vi "host.vi"() -> ()   [LabVIEW 2018]
uses:
  dll/NewTmMdsSaveLoad.dll
  epics dll/JtextEPICSforNewTM.dll
  <vilib>/rvi/interface/nirviOpenFPGA/nirviOpenFPGA.xnode
  <vilib>/FPGAPlugInAG/PCI-7813R/niLvFpga_Open_PCI-7813R.vi
  <vilib>/rvi/interface/common/dynamic/niFpgaDynamicAddResources.vi
  <vilib>/rvi/interface/nirviReadWriteControl/nirviReadWriteControl.xnode
  NiFpgaLv.dll
  <vilib>/Utility/error.llb/Error Cluster From Error Code.vi
  <vilib>/rvi/interface/Simulation/niFpgaSimulationCallBeginRW.vi
  <vilib>/rvi/errors/niLvFpgaAdjustHostInterfaceError.vi
  <vilib>/rvi/interface/nirviMethod/nirviMethod.xnode
  <vilib>/FPGAPlugInAG/Dynamic/niLvFpga_Run_Dynamic.vi
panel:
  in  "have run":enum32{"选项卡 1", "选项卡 2", "选项卡 3"}(tab)
  out "hr 1":T1
  out "hr 2":T2
  out "hr 3":T3
  in  "默认night":T1
  in  "禁用Shutup":bool
  in  "禁用Trigger":bool
  in  "be running":enum32{"选项卡 1", "选项卡 2", "选项卡 3"}(tab)
  out "lvht 1":T1
  out "lvht 2":T2
  out "lvht 3":T3
  out "act 3":bool[](array[boolean])
  out "act 2":bool[](array[boolean])
  out "act 1":bool[](array[boolean])
  out "width 3":i32[](array[numeric])
  out "begin 3":i32[](array[numeric])
  out "width 2":i32[](array[numeric])
  out "width 1":i32[](array[numeric])
  out "begin 2":i32[](array[numeric])
  out "begin 1":i32[](array[numeric])
  in  "Abort":bool
  in  "Apply":bool
  in  "最大通道数量":enum16{"96", "192", "288"}(ring)
  out "最大值":u32
  out "width":i32[](array[numeric])
  out "begin":i32[](array[numeric])
  in  "Debug":bool
  in  "Config":bool
  in  "Go":bool
  out "pv=0":bool
  out "ab":bool
  out "ShutUp":bool
  out "Ready":bool
  out "stop":bool
  out "running":bool
  out "TM state":string
  in  "pvName":string="ST:GLOBAL:CTRLSTATE"
  out "错误输出":errorcluster
  out "pv失败":bool
  in  "PV":i32=-666
  in  "Shot Number":i32
  in  "tag":string="\\NEW_TM_SET"
  in  "tree name":string="jtext"
  in  "host ip":string="192.168.1.1"
  in  "修改":T4
  in  "Mdsplus":bool
  in  "Import":path
  in  "Import":bool
  in  "Export Base Path":path
  in  "Export name":string
  in  "初始化":bool
  in  "export":bool
  in  "修改":bool
  in  "修改通道选择":enum16{"1", "2", "3", "4"}(ring)
  out "act":bool[](array[boolean])
  out "title":string[](array[string])
  out "start":dbl[](array[numeric])
  out "lenght":dbl[](array[numeric])
  out "detail":string[](array[string])
  # "be running"
  # "have run"
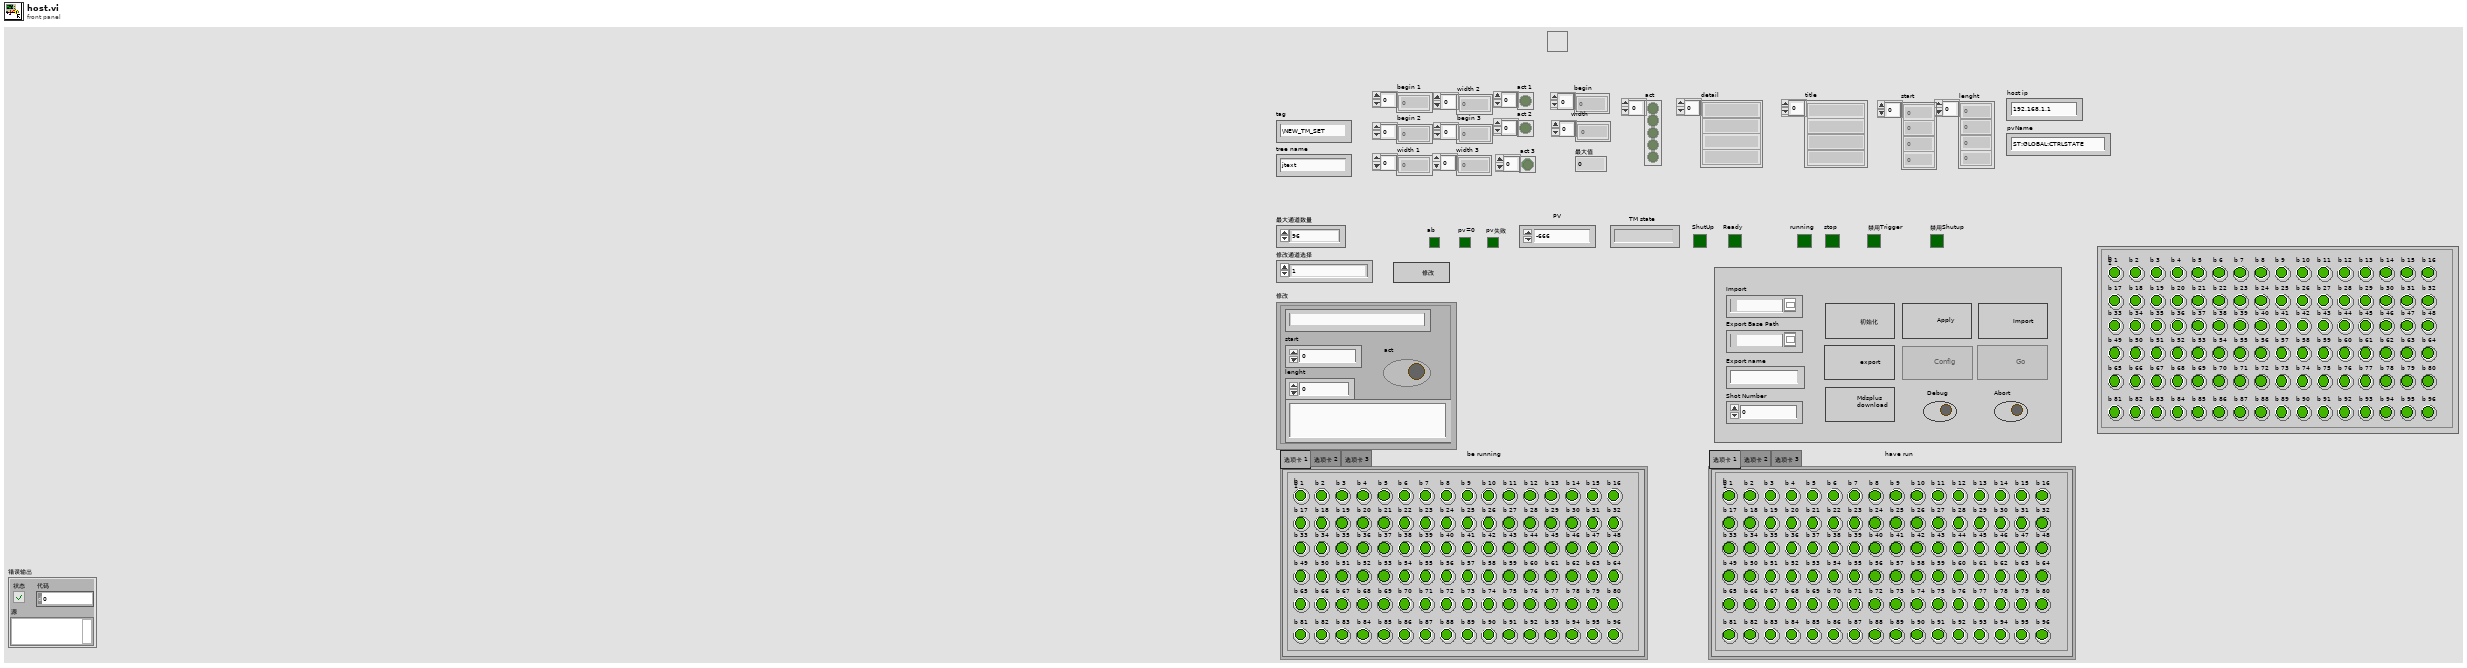
[diagram p1: front panel]
types:
  T1 = cluster{"b 1":bool, "b 2":bool, "b 3":bool, "b 4":bool, "b 5":bool, "b 6":bool, "b 7":bool, "b 8":bool, "b 9":bool, "b 10":bool, "b 11":bool, "b 12":bool, "b 13":bool, "b 14":bool, "b 15":bool, "b 16":bool, "b 17":bool, "b 18":bool, "b 19":bool, "b 20":bool, "b 21":bool, "b 22":bool, "b 23":bool, "b 24":bool, "b 25":bool, "b 26":bool, "b 27":bool, "b 28":bool, "b 29":bool, "b 30":bool, "b 31":bool, "b 32":bool, "b 33":bool, "b 34":bool, "b 35":bool, "b 36":bool, "b 37":bool, "b 38":bool, "b 39":bool, "b 40":bool, "b 41":bool, "b 42":bool, "b 43":bool, "b 44":bool, "b 45":bool, "b 46":bool, "b 47":bool, "b 48":bool, "b 49":bool, "b 50":bool, "b 51":bool, "b 52":bool, "b 53":bool, "b 54":bool, "b 55":bool, "b 56":bool, "b 57":bool, "b 58":bool, "b 59":bool, "b 60":bool, "b 61":bool, "b 62":bool, "b 63":bool, "b 64":bool, "b 65":bool, "b 66":bool, "b 67":bool, "b 68":bool, "b 69":bool, "b 70":bool, "b 71":bool, "b 72":bool, "b 73":bool, "b 74":bool, "b 75":bool, "b 76":bool, "b 77":bool, "b 78":bool, "b 79":bool, "b 80":bool, "b 81":bool, "b 82":bool, "b 83":bool, "b 84":bool, "b 85":bool, "b 86":bool, "b 87":bool, "b 88":bool, "b 89":bool, "b 90":bool, "b 91":bool, "b 92":bool, "b 93":bool, "b 94":bool, "b 95":bool, "b 96":bool}
  T2 = cluster{"b 97":bool, "b 98":bool, "b 99":bool, "b 100":bool, "b 101":bool, "b 102":bool, "b 103":bool, "b 104":bool, "b 105":bool, "b 106":bool, "b 107":bool, "b 108":bool, "b 109":bool, "b 110":bool, "b 111":bool, "b 112":bool, "b 113":bool, "b 114":bool, "b 115":bool, "b 116":bool, "b 117":bool, "b 118":bool, "b 119":bool, "b 120":bool, "b 121":bool, "b 122":bool, "b 123":bool, "b 124":bool, "b 125":bool, "b 126":bool, "b 127":bool, "b 128":bool, "b 129":bool, "b 130":bool, "b 131":bool, "b 132":bool, "b 133":bool, "b 134":bool, "b 135":bool, "b 136":bool, "b 137":bool, "b 138":bool, "b 139":bool, "b 140":bool, "b 141":bool, "b 142":bool, "b 143":bool, "b 144":bool, "b 145":bool, "b 146":bool, "b 147":bool, "b 148":bool, "b 149":bool, "b 150":bool, "b 151":bool, "b 152":bool, "b 153":bool, "b 154":bool, "b 155":bool, "b 156":bool, "b 157":bool, "b 158":bool, "b 159":bool, "b 160":bool, "b 161":bool, "b 162":bool, "b 163":bool, "b 164":bool, "b 165":bool, "b 166":bool, "b 167":bool, "b 168":bool, "b 169":bool, "b 170":bool, "b 171":bool, "b 172":bool, "b 173":bool, "b 174":bool, "b 175":bool, "b 176":bool, "b 177":bool, "b 178":bool, "b 179":bool, "b 180":bool, "b 181":bool, "b 182":bool, "b 183":bool, "b 184":bool, "b 185":bool, "b 186":bool, "b 187":bool, "b 188":bool, "b 189":bool, "b 190":bool, "b 191":bool, "b 192":bool}
  T3 = cluster{"b 193":bool, "b 194":bool, "b 195":bool, "b 196":bool, "b 197":bool, "b 198":bool, "b 199":bool, "b 200":bool, "b 201":bool, "b 202":bool, "b 203":bool, "b 204":bool, "b 205":bool, "b 206":bool, "b 207":bool, "b 208":bool, "b 209":bool, "b 210":bool, "b 211":bool, "b 212":bool, "b 213":bool, "b 214":bool, "b 215":bool, "b 216":bool, "b 217":bool, "b 218":bool, "b 219":bool, "b 220":bool, "b 221":bool, "b 222":bool, "b 223":bool, "b 224":bool, "b 225":bool, "b 226":bool, "b 227":bool, "b 228":bool, "b 229":bool, "b 230":bool, "b 231":bool, "b 232":bool, "b 233":bool, "b 234":bool, "b 235":bool, "b 236":bool, "b 237":bool, "b 238":bool, "b 239":bool, "b 240":bool, "b 241":bool, "b 242":bool, "b 243":bool, "b 244":bool, "b 245":bool, "b 246":bool, "b 247":bool, "b 248":bool, "b 249":bool, "b 250":bool, "b 251":bool, "b 252":bool, "b 253":bool, "b 254":bool, "b 255":bool, "b 256":bool, "b 257":bool, "b 258":bool, "b 259":bool, "b 260":bool, "b 261":bool, "b 262":bool, "b 263":bool, "b 264":bool, "b 265":bool, "b 266":bool, "b 267":bool, "b 268":bool, "b 269":bool, "b 270":bool, "b 271":bool, "b 272":bool, "b 273":bool, "b 274":bool, "b 275":bool, "b 276":bool, "b 277":bool, "b 278":bool, "b 279":bool, "b 280":bool, "b 281":bool, "b 282":bool, "b 283":bool, "b 284":bool, "b 285":bool, "b 286":bool, "b 287":bool, "b 288":bool}
  T4 = cluster{"title":string, "act":bool, "start":dbl, "lenght":dbl, "detail":string}
  T5 = enum16{"open", "open or create", "create or replace", "create", "open (read-only)"}
  T6 = cluster{string[], bool[], dbl[], dbl[], string[]}
  T7 = enum16{"open", "replace", "create", "open or create", "replace or create", "replace or create with confirmation"}
  T8 = cluster{"字符串":string, "act":bool, "start":dbl, "lenght":dbl, "详细信息":string}
  T9 = enum8{"Enabled", "Disabled", "Disabled and Grayed Out"}
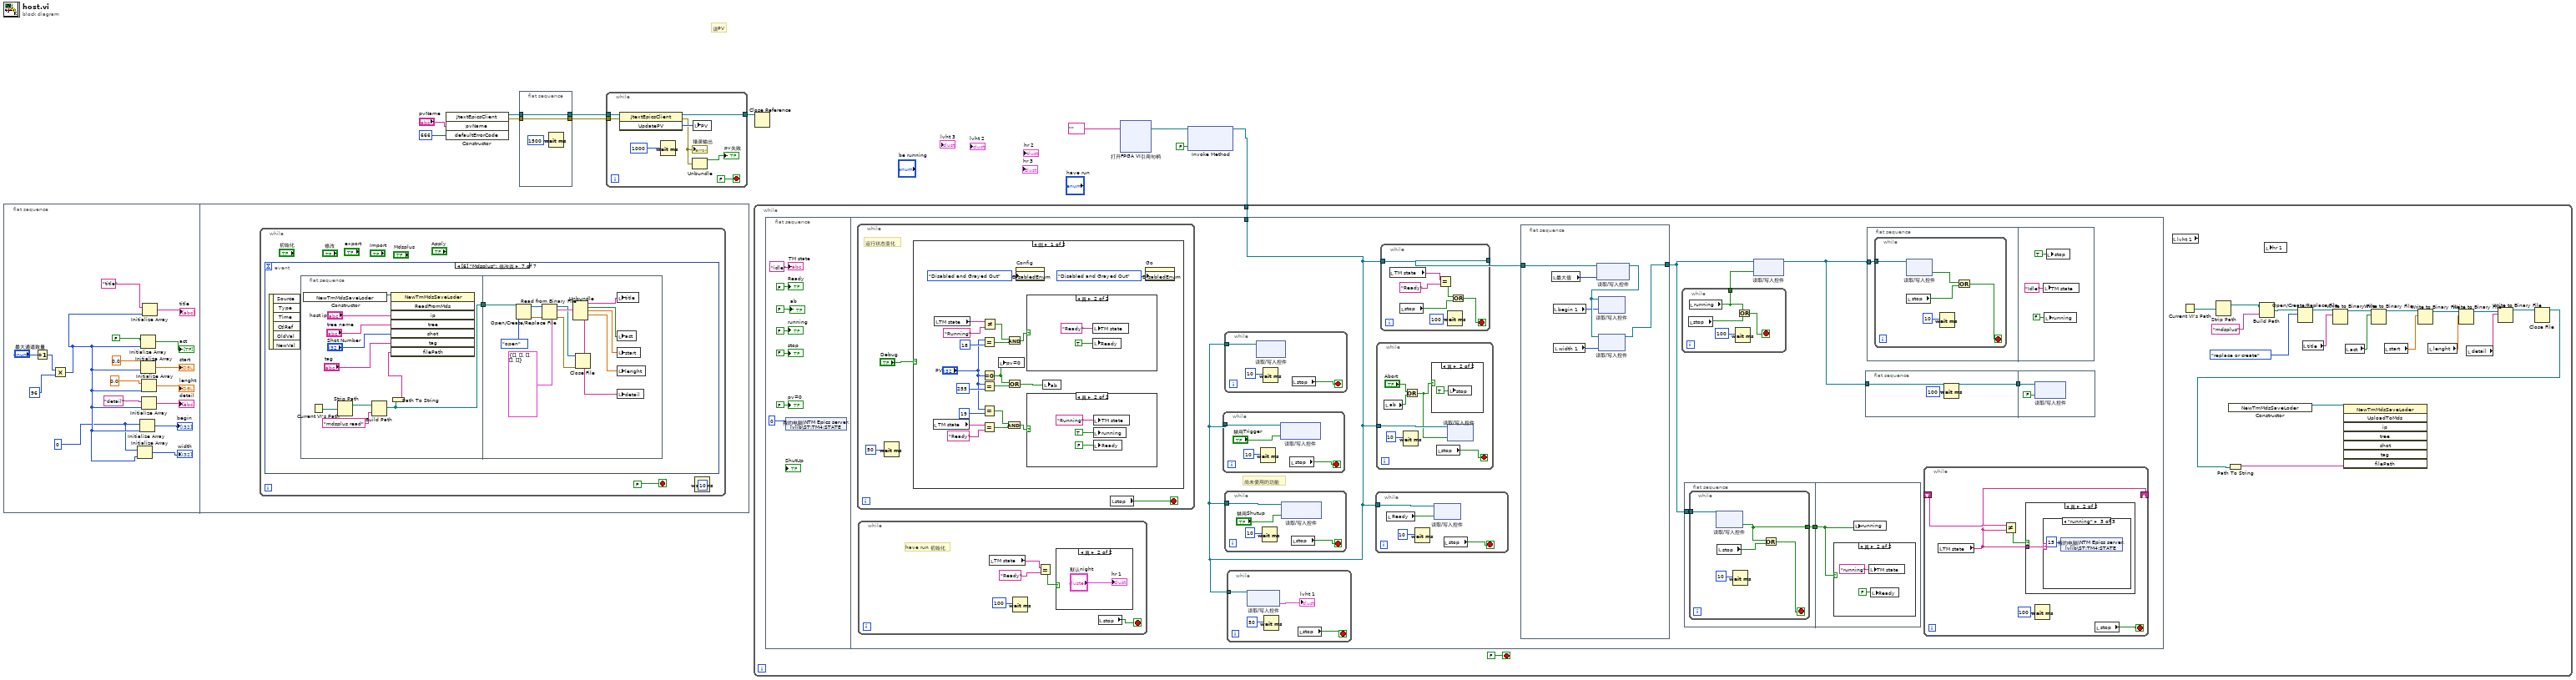
[diagram p0: block diagram]
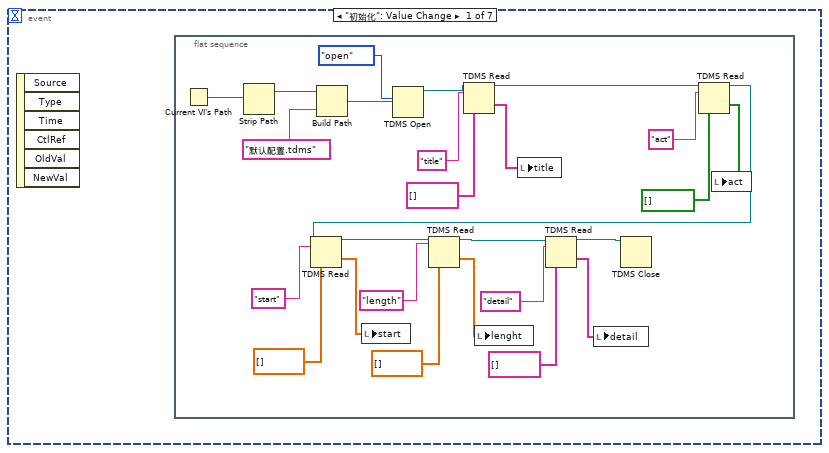
[diagram p2: hidden frame]
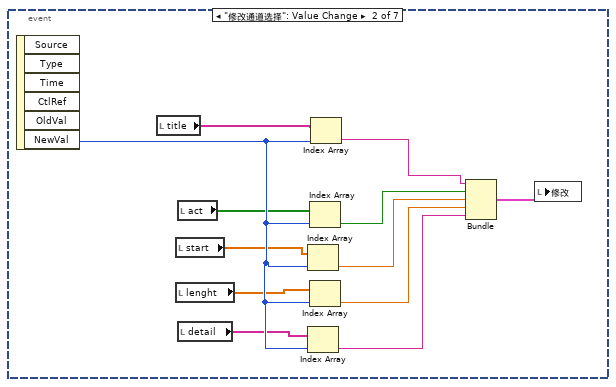
[diagram p3: hidden frame]
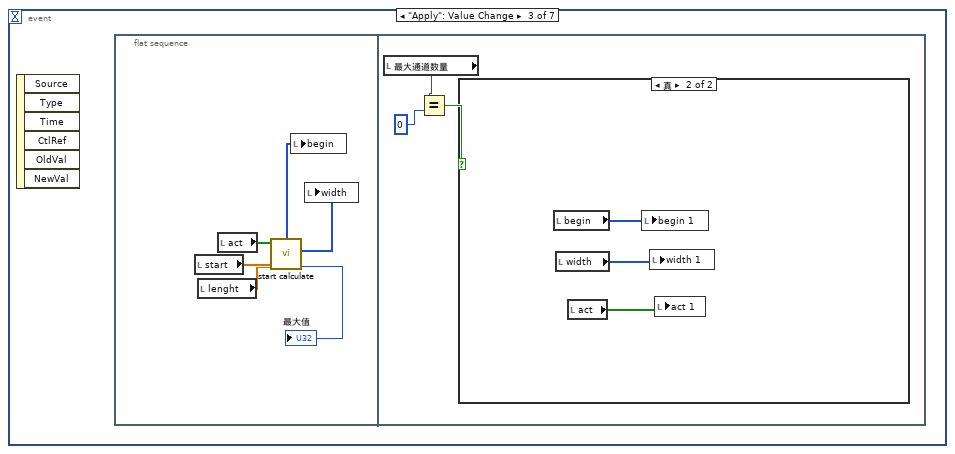
[diagram p4: hidden frame]
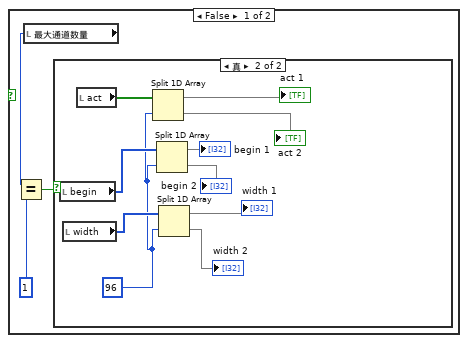
[diagram p5: hidden frame]
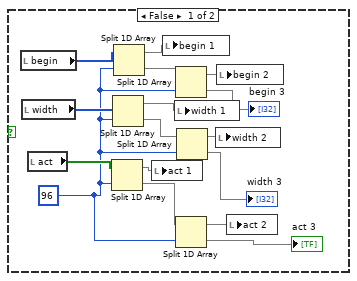
[diagram p6: hidden frame]
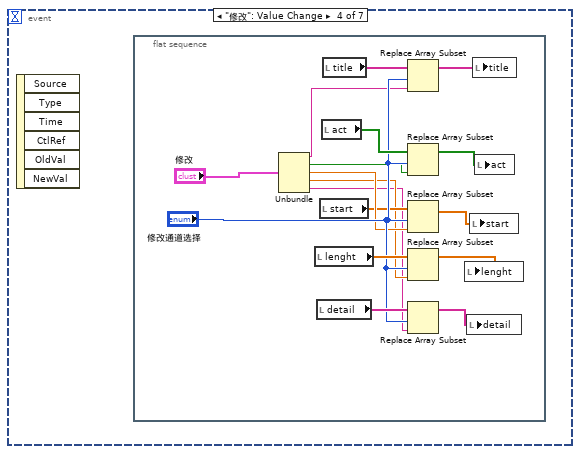
[diagram p7: hidden frame]
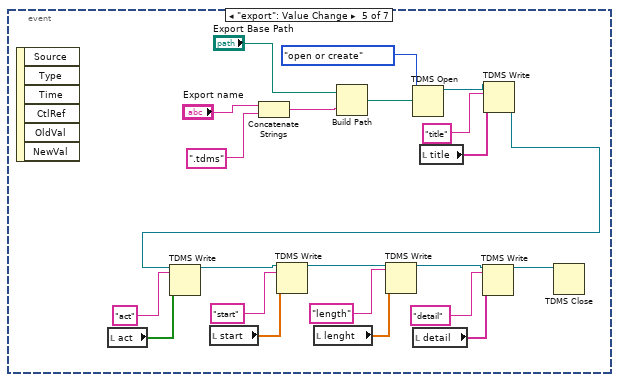
[diagram p8: hidden frame]
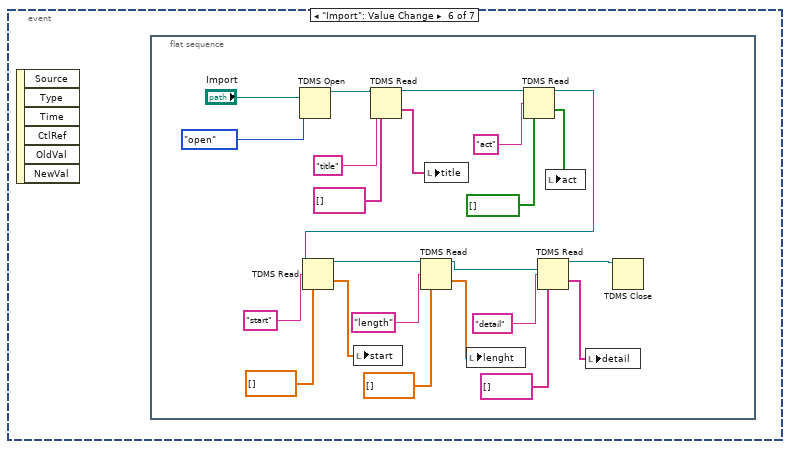
[diagram p9: hidden frame]
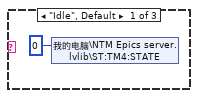
[diagram p11: hidden frame]
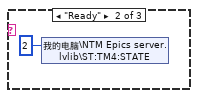
[diagram p12: hidden frame]
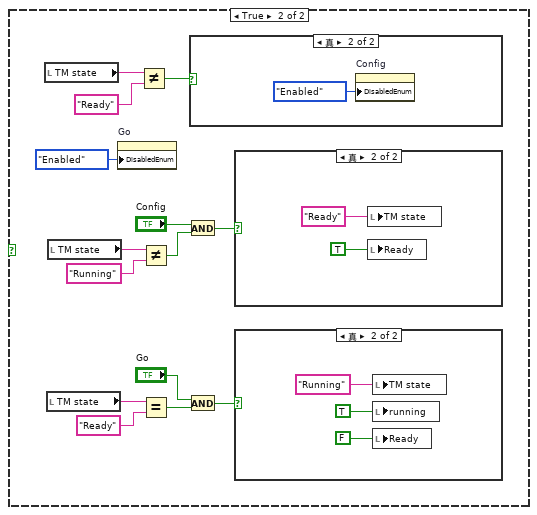
[diagram p18: hidden frame]
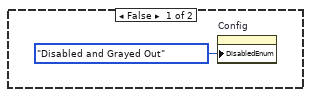
[diagram p19: hidden frame]
diagram:
  # "读PV"
  n1 = flat-sequence {
    frame #0 {
      w12 = 0
      n2 = Increment(x="最大通道数量") -> (x+1=w16:enum16{"96", "192", "288"})
      n3 = Multiply(x=w16, y=96) -> (x*y=w15:i32)
      n4 = Initialize Array(w12, w15) -> (→"width":i32[])
      n5 = Initialize Array(w12, w15) -> (→"begin":i32[])
      n6 = Initialize Array(FALSE, w15) -> (→"act":bool[])
      n7 = Initialize Array(0.0, w15) -> (→"start":dbl[])
      n8 = Initialize Array(0.0, w15) -> (→"lenght":dbl[])
      n9 = Initialize Array("detail", w15) -> (→"detail":string[])
      n10 = Initialize Array("title", w15) -> (→"title":string[])
    }
    frame #1 {
      n11 = while {
        stop <- FALSE stop-if-true
        n12 = event shown="[6] \"Mdsplus\": 值改变" {
          selector: _ -> [_ _ _ _ _ _ _]
          dyn-events: _ -> [_ _ _ _ _ _ _]
          timeout: _ -> [_ _ _ _ _ _ _]
          event "初始化": Value Change {
            n13 = event-data() -> ()  [unwired: 1 in, 6 out]
            n14 = flat-sequence {
              frame #0 {
                n15 = Current VI's Path() -> (path=w56:path)
                n16 = Strip Path(path=w56) -> (stripped path=w55:path)  [unwired: 1 out]
                n17 = Build Path(base path=w55, name or relative path="默认配置.tdms") -> (appended path=w54:path)
                n18 = TDMS Open(10:T5."open" ("操作(0:open)"), 11:w54) -> (3:w53:refnum<k34>)  [unwired: 5 in, 1 out]
                n19 = TDMS Read(0:w53, 5:"title" ("通道名输入（无标题）"), 12:string[] []) -> (4:w36:refnum<k34>, 10:w49:string[])  [unwired: 5 in, 4 out]
                n20 = local write "title"(w49) -> ()
                n21 = TDMS Read(0:w36, 5:"act" ("通道名输入（无标题）"), 12:bool[] []) -> (4:w46:refnum<k34>, 10:w41:bool[])  [unwired: 5 in, 4 out]
                n22 = TDMS Read(0:w46, 5:"start" ("通道名输入（无标题）"), 12:dbl[] []) -> (4:w45:refnum<k34>, 10:w39:dbl[])  [unwired: 5 in, 4 out]
                n23 = local write "start"(w39) -> ()
                n24 = TDMS Read(0:w45, 5:"length" ("通道名输入（无标题）"), 12:dbl[] []) -> (4:w44:refnum<k34>, 10:w37:dbl[])  [unwired: 5 in, 4 out]
                n25 = local write "lenght"(w37) -> ()
                n26 = TDMS Read(0:w44, 5:"detail" ("通道名输入（无标题）"), 12:string[] []) -> (4:w43:refnum<k34>, 10:w48:string[])  [unwired: 5 in, 4 out]
                n27 = local write "detail"(w48) -> ()
                n28 = TDMS Close(11:w43) -> ()  [unwired: 1 in, 2 out]
                n29 = local write "act"(w41) -> ()
              }
            }
          }
          event "修改通道选择": Value Change {
            n30 = event-data() -> ("NewVal"=w67:enum16{"1", "2", "3", "4"})  [unwired: 1 in, 5 out]
            n31 = local read "title"() -> (w68:string[])
            n32 = local read "start"() -> (w64:dbl[])
            n33 = local read "lenght"() -> (w65:dbl[])
            n34 = local read "act"() -> (w63:bool[])
            n35 = local read "detail"() -> (w66:string[])
            n36 = Index Array(array=w64, index=w67) -> (element=w61:dbl)
            n37 = Index Array(array=w66, index=w67) -> (element=w59:string)
            n38 = Index Array(array=w63, index=w67) -> (element=w62:bool)
            n39 = Index Array(array=w65, index=w67) -> (element=w60:dbl)
            n40 = Index Array(array=w68, index=w67) -> (element=w58:string)
            n41 = Bundle("字符串"=w58, "act"=w62, "start"=w61, "lenght"=w60, "详细信息"=w59) -> (w57:T8)  [unwired: 1 in]
            n42 = local write "修改"(w57) -> ()
          }
          event "Apply": Value Change {
            n43 = event-data() -> ()  [unwired: 1 in, 6 out]
            n44 = flat-sequence {
              frame #0 {
                n45 = local read "start"() -> (w73:dbl[])
                n46 = local read "lenght"() -> (w72:dbl[])
                n47 = local read "act"() -> (w71:bool[])
                n48 = call "start calculate.vi"("lenght"=w72, "start"=w73, "act"=w71) -> ("最大值"=→"最大值":i32, "width"=w69:i32[], "begin"=w70:i32[])  [unwired: 6 in]
                n49 = local write "begin"(w70) -> ()
                n50 = local write "width"(w69) -> ()
              }
              frame #1 {
                n51 = local read "最大通道数量"() -> (w76:enum16{"96", "192", "288"})
                n52 = Equal?(x=w76, y=0) -> (x = y?=w75:bool)
                n53 = case shown="真" w75 {
                  frame False {
                    n54 = local read "最大通道数量"() -> (w80:enum16{"96", "192", "288"})
                    n55 = Equal?(x=w80, y=1) -> (x = y?=w78:bool)
                    n56 = case shown="真" w78 {
                      frame False {
                        w84 = 96
                        n57 = local read "begin"() -> (w96:i32[])
                        n58 = local read "width"() -> (w95:i32[])
                        n59 = local read "act"() -> (w86:bool[])
                        n60 = Split 1D Array(array=w86, index=w84) -> (first subarray=w83:bool[], second subarray=w85:bool[])
                        n61 = Split 1D Array(array=w95, index=w84) -> (first subarray=w90:i32[], second subarray=w93:i32[])
                        n62 = Split 1D Array(array=w96, index=w84) -> (first subarray=w92:i32[], second subarray=w94:i32[])
                        n63 = local write "act 1"(w83) -> ()
                        n64 = local write "begin 1"(w92) -> ()
                        n65 = local write "width 1"(w90) -> ()
                        n66 = Split 1D Array(array=w94, index=w84) -> (first subarray=w91:i32[], second subarray=→"begin 3":i32[])
                        n67 = Split 1D Array(array=w85, index=w84) -> (first subarray=w82:bool[], second subarray=→"act 3":bool[])
                        n68 = Split 1D Array(array=w93, index=w84) -> (first subarray=w89:i32[], second subarray=→"width 3":i32[])
                        n69 = local write "width 2"(w89) -> ()
                        n70 = local write "begin 2"(w91) -> ()
                        n71 = local write "act 2"(w82) -> ()
                      }
                      frame True {
                        w100 = 96
                        n72 = local read "begin"() -> (w106:i32[])
                        n73 = local read "width"() -> (w105:i32[])
                        n74 = local read "act"() -> (w99:bool[])
                        n75 = Split 1D Array(array=w99, index=w100) -> (first subarray=→"act 1":bool[], second subarray=→"act 2":bool[])
                        n76 = Split 1D Array(array=w106, index=w100) -> (first subarray=→"begin 1":i32[], second subarray=→"begin 2":i32[])
                        n77 = Split 1D Array(array=w105, index=w100) -> (first subarray=→"width 1":i32[], second subarray=→"width 2":i32[])
                      }
                    }
                  }
                  frame True {
                    n78 = local read "begin"() -> (w109:i32[])
                    n79 = local read "width"() -> (w108:i32[])
                    n80 = local read "act"() -> (w107:bool[])
                    n81 = local write "begin 1"(w109) -> ()
                    n82 = local write "width 1"(w108) -> ()
                    n83 = local write "act 1"(w107) -> ()
                  }
                }
              }
            }
          }
          event "修改": Value Change {
            n84 = event-data() -> ()  [unwired: 1 in, 6 out]
            n85 = flat-sequence {
              frame #0 {
                n86 = Unbundle("修改") -> ("title"=w121:string, "act"=w115:bool, "start"=w114:dbl, "lenght"=w112:dbl, "detail"=w111:string)
                n87 = local read "lenght"() -> (w124:dbl[])
                n88 = local read "detail"() -> (w123:string[])
                n89 = local read "start"() -> (w113:dbl[])
                n90 = local read "act"() -> (w125:bool[])
                n91 = local read "title"() -> (w126:string[])
                n92 = Replace Array Subset(array=w126, new element=w121, index="修改通道选择") -> (w120:string[])
                n93 = Replace Array Subset(array=w125, new element=w115, index="修改通道选择") -> (w119:bool[])
                n94 = Replace Array Subset(array=w113, new element=w114, index="修改通道选择") -> (w110:dbl[])
                n95 = Replace Array Subset(array=w124, new element=w112, index="修改通道选择") -> (w118:dbl[])
                n96 = Replace Array Subset(array=w123, new element=w111, index="修改通道选择") -> (w117:string[])
                n97 = local write "lenght"(w118) -> ()
                n98 = local write "detail"(w117) -> ()
                n99 = local write "start"(w110) -> ()
                n100 = local write "title"(w120) -> ()
                n101 = local write "act"(w119) -> ()
              }
            }
          }
          event "export": Value Change {
            n102 = event-data() -> ()  [unwired: 1 in, 6 out]
            n103 = local read "act"() -> (w144:bool[])
            n104 = local read "start"() -> (w143:dbl[])
            n105 = Concatenate Strings("Export name", ".tdms" ("字符串")) -> (w134:string)
            n106 = local read "lenght"() -> (w142:dbl[])
            n107 = Build Path(base path="Export Base Path", name or relative path=w134) -> (appended path=w148:path)
            n108 = TDMS Open(10:T5."open or create" ("操作(0:open)"), 11:w148) -> (3:w146:refnum<k34>)  [unwired: 5 in, 1 out]
            n109 = local read "detail"() -> (w141:string[])
            n110 = local read "title"() -> (w145:string[])
            n111 = TDMS Write(0:w146, 5:"title" ("通道名输入（无标题）"), 9:w145) -> (4:w132:refnum<k34>)  [unwired: 3 in, 3 out]
            n112 = TDMS Write(0:w132, 5:"act" ("通道名输入（无标题）"), 9:w144) -> (4:w140:refnum<k34>)  [unwired: 3 in, 3 out]
            n113 = TDMS Write(0:w140, 5:"start" ("通道名输入（无标题）"), 9:w143) -> (4:w139:refnum<k34>)  [unwired: 3 in, 3 out]
            n114 = TDMS Write(0:w139, 5:"length" ("通道名输入（无标题）"), 9:w142) -> (4:w138:refnum<k34>)  [unwired: 3 in, 3 out]
            n115 = TDMS Write(0:w138, 5:"detail" ("通道名输入（无标题）"), 9:w141) -> (4:w137:refnum<k34>)  [unwired: 3 in, 3 out]
            n116 = TDMS Close(11:w137) -> ()  [unwired: 1 in, 2 out]
          }
          event "Import": Value Change {
            n117 = event-data() -> ()  [unwired: 1 in, 6 out]
            n118 = flat-sequence {
              frame #0 {
                n119 = TDMS Open(10:T5."open" ("操作(0:open)"), 11:"Import") -> (3:w171:refnum<k34>)  [unwired: 5 in, 1 out]
                n120 = TDMS Read(0:w171, 7:"title" ("通道名输入（无标题）"), 12:string[] []) -> (4:w149:refnum<k34>, 10:w170:string[])  [unwired: 5 in, 4 out]
                n121 = local write "title"(w170) -> ()
                n122 = TDMS Read(0:w149, 7:"act" ("通道名输入（无标题）"), 12:bool[] []) -> (4:w168:refnum<k34>, 10:w164:bool[])  [unwired: 5 in, 4 out]
                n123 = TDMS Read(0:w168, 7:"start" ("通道名输入（无标题）"), 12:dbl[] []) -> (4:w167:refnum<k34>, 10:w163:dbl[])  [unwired: 5 in, 4 out]
                n124 = local write "start"(w163) -> ()
                n125 = TDMS Read(0:w167, 7:"length" ("通道名输入（无标题）"), 12:dbl[] []) -> (4:w166:refnum<k34>, 10:w162:dbl[])  [unwired: 5 in, 4 out]
                n126 = local write "lenght"(w162) -> ()
                n127 = TDMS Read(0:w166, 7:"detail" ("通道名输入（无标题）"), 12:string[] []) -> (4:w165:refnum<k34>, 10:w169:string[])  [unwired: 5 in, 4 out]
                n128 = local write "act"(w164) -> ()
                n129 = local write "detail"(w169) -> ()
                n130 = TDMS Close(11:w165) -> ()  [unwired: 1 in, 2 out]
              }
            }
          }
          event "Mdsplus": Value Change {
            n131 = event-data() -> ()  [unwired: 1 in, 6 out]
            n132 = flat-sequence {
              tunnel: [w174] -> w172
              tunnel: w172 -> [w195]
              frame #0 {
                n133 = constructor class="NewTmMdsSaveLoder"() -> (reference out=w182:refnum<k24>)  [unwired: 3 in, 2 out]
                n134 = Current VI's Path() -> (path=w176:path)
                n135 = Strip Path(path=w176) -> (stripped path=w173:path)  [unwired: 1 out]
                n136 = Build Path(base path=w173, name or relative path="mdsplus read" ("名称或相对路径")) -> (appended path=w174:path)
                n137 = Path To String(path=w174) -> (string=w175:string)
                n138 = invoke class="NewTmMdsSaveLoder" method="ReadFromMds"(reference=w182, "ip"="host ip", "tree"="tree name", "shot"="Shot Number", "tag"="tag", "filePath"=w175) -> ()  [unwired: 2 in, 8 out]
              }
              frame #1 {
                n139 = Open/Create/Replace File(file path (use dialog)=w195, operation (0:open)=T7."open" ("操作(0:open)")) -> (refnum out=w193:refnum<file>, error out=w194:errorcluster)  [unwired: 4 in, 1 out]
                n140 = Read from Binary File(5:T6 {[], [], [], [], []}, 8:w194, 11:w193) -> (0:w187:errorcluster, 2:w190:T6, 3:w188:refnum<file>)  [unwired: 3 in, 1 out]
                n141 = Unbundle(w190) -> (w189:string[], w186:bool[], w185:dbl[], w184:dbl[], w183:string[])
                n142 = Close File(refnum=w188, error in=w187) -> ()  [unwired: 2 out]
                n143 = local write "title"(w189) -> ()
                n144 = local write "act"(w186) -> ()
                n145 = local write "start"(w185) -> ()
                n146 = local write "lenght"(w184) -> ()
                n147 = local write "detail"(w183) -> ()
              }
            }
          }
        }
        n148 = Wait (ms)(milliseconds to wait=u32 10 ("等待时间（毫秒）")) -> ()  [unwired: 1 out]
      }
    }
  }
  n149 = constructor class="JtextEpicsClient"("pvName"="pvName", "defaultErrorCode"=666) -> (reference out=w9:refnum<k24>, error out=w11:errorcluster)  [unwired: 3 in, 3 out]
  n150 = flat-sequence {
    tunnel: [w197] -> w8
    tunnel: w9 -> [w197]
    tunnel: [w196] -> w10
    tunnel: w11 -> [w196]
    frame #0 {
      n151 = Wait (ms)(milliseconds to wait=u32 1500 ("等待时间（毫秒）")) -> ()  [unwired: 1 out]
    }
  }
  n152 = while {
    tunnel: w8 -> [w205]
    tunnel: [w203] -> w7
    tunnel: w10 -> [w202]
    stop <- FALSE stop-if-true
    n153 = invoke on="调用节点" class="JtextEpicsClient" method="UpdatePV"(reference=w205, error in=w202) -> (reference out=w203:refnum<k24>, error out=w201:errorcluster, "UpdatePV"=w204:i32)  [unwired: 1 in]
    "错误输出" <- w201
    n154 = Wait (ms)(milliseconds to wait=u32 1000 ("等待时间（毫秒）")) -> ()  [unwired: 1 out]
    n155 = Unbundle(w201) -> ("status"=→"pv失败":bool)  [unwired: 2 out]
    n156 = local write "PV"(w204) -> ()
  }
  n157 = Close Reference(reference=w7) -> ()  [unwired: 1 in, 1 out]
  n158 = xnode "打开FPGA VI引用句柄"("资源名称"=tag "") -> ("FPGA VI引用输出"=w3:refnum<k20>)  [unwired: 1 in, 1 out]
  n159 = xnode "Invoke Method"("FPGA VI引用输入"=w3, "结束前等待(F)"=FALSE) -> ("FPGA VI引用输出"=w2:refnum<k20>)  [unwired: 1 in, 1 out]
  n160 = while {
    tunnel: w2 -> [w226]
    stop <- FALSE stop-if-true
    n161 = flat-sequence {
      tunnel: w226 -> [w240]
      frame #0 {
        n162 = shared-variable "我的电脑\\NTM Epics server.lvlib\\ST:TM4:STATE"(0 ("ST:TM4:STATE")) -> ()  [unwired: 1 in, 1 out]
        "TM state" <- "idle" ("TM state")
        "Ready" <- FALSE ("Ready")
        "ab" <- FALSE ("ab")
        "running" <- FALSE ("running")
        "stop" <- FALSE ("stop")
        "pv=0" <- FALSE ("pv=0")
      }
      frame #1 {
        # "尚未使用的功能"
        n163 = while {
          stop <- w323 stop-if-true
          # "运行状态变化"
          n164 = Wait (ms)(milliseconds to wait=u32 50 ("等待时间（毫秒）")) -> ()  [unwired: 1 out]
          n165 = case shown="假" "Debug" {
            frame False {
              n166 = local read "TM state"() -> (w344:string)
              n167 = local read "TM state"() -> (w332:string)
              n168 = Equal?(x="PV", y=18) -> (x = y?=w334:bool)
              n169 = Equal To 0?(x="PV") -> (x = 0?=w327:bool)
              n170 = Equal?(x="PV", y=255) -> (x = y?=w329:bool)
              n171 = Equal?(x="PV", y=19) -> (x = y?=w340:bool)
              n172 = Equal?(x=w344, y="Ready") -> (x = y?=w342:bool)
              n173 = Not Equal?(x=w332, y="Running") -> (x != y?=w331:bool)
              n174 = local write "pv=0"(w327) -> ()
              n175 = And(x=w340, y=w342) -> (x .and. y?=w341:bool)
              n176 = And(x=w331, y=w334) -> (x .and. y?=w335:bool)
              n177 = Or(x=w327, y=w329) -> (x .or. y?=w326:bool)
              n178 = property on="Config" class="Bool"("DisabledEnum"=T9."Disabled and Grayed Out" ("禁用")) -> ()  [unwired: 2 in, 2 out]
              n179 = case shown="真" w335 {
                frame False {
                }
                frame True {
                  n180 = local write "TM state"("Ready" ("TM state")) -> ()
                  n181 = local write "Ready"(TRUE ("running")) -> ()
                }
              }
              n182 = case shown="真" w341 {
                frame False {
                }
                frame True {
                  n183 = local write "TM state"("Running" ("TM state")) -> ()
                  n184 = local write "running"(TRUE ("running")) -> ()
                  n185 = local write "Ready"(FALSE ("running")) -> ()
                }
              }
              n186 = local write "ab"(w326) -> ()
              n187 = property on="Go" class="Bool"("DisabledEnum"=T9."Disabled and Grayed Out" ("禁用")) -> ()  [unwired: 2 in, 2 out]
            }
            frame True {
              n188 = local read "TM state"() -> (w356:string)
              n189 = local read "TM state"() -> (w363:string)
              n190 = local read "TM state"() -> (w351:string)
              n191 = property on="Go" class="Bool"("DisabledEnum"=T9."Enabled" ("禁用")) -> ()  [unwired: 2 in, 2 out]
              n192 = Not Equal?(x=w356, y="Ready") -> (x != y?=w355:bool)
              n193 = Not Equal?(x=w351, y="Running") -> (x != y?=w350:bool)
              n194 = Equal?(x=w363, y="Ready") -> (x = y?=w361:bool)
              n195 = And(x="Config", y=w350) -> (x .and. y?=w354:bool)
              n196 = And(x="Go", y=w361) -> (x .and. y?=w359:bool)
              n197 = case shown="真" w355 {
                frame False {
                  n198 = property on="Config" class="Bool"("DisabledEnum"=T9."Disabled and Grayed Out" ("禁用")) -> ()  [unwired: 2 in, 2 out]
                }
                frame True {
                  n199 = property on="Config" class="Bool"("DisabledEnum"=T9."Enabled" ("禁用")) -> ()  [unwired: 2 in, 2 out]
                }
              }
              n200 = case shown="真" w354 {
                frame False {
                }
                frame True {
                  n201 = local write "TM state"("Ready" ("TM state")) -> ()
                  n202 = local write "Ready"(TRUE ("running")) -> ()
                }
              }
              n203 = case shown="真" w359 {
                frame False {
                }
                frame True {
                  n204 = local write "TM state"("Running" ("TM state")) -> ()
                  n205 = local write "running"(TRUE ("running")) -> ()
                  n206 = local write "Ready"(FALSE ("running")) -> ()
                }
              }
            }
          }
          n207 = local read "stop"() -> (w323:bool)
        }
        n208 = while {
          stop <- w288 stop-if-true
          # "have run 初始化"
          n209 = local read "TM state"() -> (w286:string)
          n210 = Wait (ms)(milliseconds to wait=u32 100 ("等待时间（毫秒）")) -> ()  [unwired: 1 out]
          n211 = Equal?(x=w286, y="Ready") -> (x = y?=w285:bool)
          n212 = case shown="真" w285 {
            frame False {
            }
            frame True {
              "hr 1" <- "默认night"
            }
          }
          n213 = local read "stop"() -> (w288:bool)
        }
        n214 = while {
          tunnel: w240 -> [w300]
          stop <- w299 stop-if-true
          n215 = Wait (ms)(milliseconds to wait=u32 10 ("等待时间（毫秒）")) -> ()  [unwired: 1 out]
          n216 = xnode "读取/写入控件"("FPGA VI引用输入"=w300, "禁用trigger"="禁用Trigger") -> ()  [unwired: 1 in, 2 out]
          n217 = local read "stop"() -> (w299:bool)
        }
        n218 = while {
          tunnel: w240 -> [w296]
          stop <- w295 stop-if-true
          n219 = Wait (ms)(milliseconds to wait=u32 10 ("等待时间（毫秒）")) -> ()  [unwired: 1 out]
          n220 = xnode "读取/写入控件"("FPGA VI引用输入"=w296, "禁用shutup"="禁用Shutup") -> ()  [unwired: 1 in, 2 out]
          n221 = local read "stop"() -> (w295:bool)
        }
        n222 = while {
          tunnel: w240 -> [w303]
          stop <- w302 stop-if-true
          n223 = xnode "读取/写入控件"("FPGA VI引用输入"=w303) -> ()  [unwired: 1 in, 3 out]
          n224 = Wait (ms)(milliseconds to wait=u32 10 ("等待时间（毫秒）")) -> ()  [unwired: 1 out]
          n225 = local read "stop"() -> (w302:bool)
        }
        n226 = while {
          tunnel: w240 -> [w293]
          stop <- w290 stop-if-true
          n227 = xnode "读取/写入控件"("FPGA VI引用输入"=w293) -> ("lvnight 1"=→"lvht 1":T1)  [unwired: 1 in, 2 out]
          n228 = Wait (ms)(milliseconds to wait=u32 50 ("等待时间（毫秒）")) -> ()  [unwired: 1 out]
          n229 = local read "stop"() -> (w290:bool)
        }
        n230 = while {
          tunnel: w240 -> [w307]
          stop <- w305 stop-if-true
          n231 = local read "Ready"() -> (w306:bool)
          n232 = Wait (ms)(milliseconds to wait=u32 10 ("等待时间（毫秒）")) -> ()  [unwired: 1 out]
          n233 = xnode "读取/写入控件"("FPGA VI引用输入"=w307, "Ready"=w306) -> ()  [unwired: 1 in, 2 out]
          n234 = local read "stop"() -> (w305:bool)
        }
        n235 = while {
          tunnel: w240 -> [w310]
          stop <- w311 stop-if-true
          n236 = local read "ab"() -> (w313:bool)
          n237 = Wait (ms)(milliseconds to wait=u32 10 ("等待时间（毫秒）")) -> ()  [unwired: 1 out]
          n238 = Or(x="Abort", y=w313) -> (x .or. y?=w309:bool)
          n239 = case shown="真" w309 {
            frame False {
            }
            frame True {
              n240 = local write "stop"(TRUE ("stop")) -> ()
            }
          }
          n241 = local read "stop"() -> (w311:bool)
          n242 = xnode "读取/写入控件"("FPGA VI引用输入"=w310, "Abort"=w309) -> ()  [unwired: 1 in, 2 out]
        }
        n243 = while {
          tunnel: w240 -> [w322]
          tunnel: [w322] -> w241
          stop <- w317 stop-if-true
          n244 = local read "TM state"() -> (w321:string)
          n245 = local read "stop"() -> (w318:bool)
          n246 = Equal?(x=w321, y="Ready") -> (x = y?=w319:bool)
          n247 = Wait (ms)(milliseconds to wait=u32 100 ("等待时间（毫秒）")) -> ()  [unwired: 1 out]
          n248 = Or(x=w319, y=w318) -> (x .or. y?=w317:bool)
        }
        n249 = flat-sequence {
          tunnel: w241 -> [w283]
          tunnel: [w278] -> w235
          frame #0 {
            n250 = local read "最大值"() -> (w282:u32)
            n251 = local read "begin 1"() -> (w280:i32[])
            n252 = local read "width 1"() -> (w279:i32[])
            n253 = xnode "读取/写入控件"("FPGA VI引用输入"=w283, "max0+1"=w282) -> ("FPGA VI引用输出"=w281:refnum<k20>)  [unwired: 1 in, 1 out]
            n254 = xnode "读取/写入控件"("FPGA VI引用输入"=w281, "begin"=w280) -> ()  [unwired: 1 in, 2 out]
            n255 = xnode "读取/写入控件"("FPGA VI引用输入"=w281, "width"=w279) -> ("FPGA VI引用输出"=w278:refnum<k20>)  [unwired: 1 in, 1 out]
          }
        }
        n256 = while {
          tunnel: [w277] -> w239
          stop <- w275 stop-if-true
          n257 = local read "stop"() -> (w276:bool)
          n258 = local read "running"() -> (w277:bool)
          n259 = Wait (ms)(milliseconds to wait=u32 100 ("等待时间（毫秒）")) -> ()  [unwired: 1 out]
          n260 = Or(x=w277, y=w276) -> (x .or. y?=w275:bool)
        }
        n261 = flat-sequence {
          tunnel: w235 -> [w256]
          tunnel: [w255] -> w238
          tunnel: w238 -> [w262]
          frame #0 {
            n262 = while {
              tunnel: w256 -> [w261]
              tunnel: [w258] -> w255
              stop <- w259 stop-if-true
              n263 = xnode "读取/写入控件"("FPGA VI引用输入"=w261) -> ("T-run"=w258:bool)  [unwired: 1 in, 2 out]
              n264 = local read "stop"() -> (w260:bool)
              n265 = Wait (ms)(milliseconds to wait=u32 10 ("等待时间（毫秒）")) -> ()  [unwired: 1 out]
              n266 = Or(x=w258, y=w260) -> (x .or. y?=w259:bool)
            }
          }
          frame #1 {
            n267 = case shown="真" w262 {
              frame False {
              }
              frame True {
                n268 = local write "TM state"("running" ("TM state")) -> ()
                n269 = local write "Ready"(FALSE ("Ready")) -> ()
              }
            }
            n270 = local write "running"(w262) -> ()
          }
        }
        n271 = xnode "读取/写入控件"("FPGA VI引用输入"=w235, "running"=w239) -> ("FPGA VI引用输出"=w236:refnum<k20>)  [unwired: 1 in, 1 out]
        n272 = flat-sequence {
          tunnel: [w251] -> w237
          tunnel: w236 -> [w251]
          tunnel: w237 -> [w254]
          frame #0 {
            n273 = Wait (ms)(milliseconds to wait=u32 100 ("等待时间（毫秒）")) -> ()  [unwired: 1 out]
          }
          frame #1 {
            n274 = xnode "读取/写入控件"("FPGA VI引用输入"=w254, "running"=FALSE) -> ()  [unwired: 1 in, 2 out]
          }
        }
        n275 = flat-sequence {
          tunnel: w236 -> [w265]
          frame #0 {
            n276 = while {
              tunnel: w265 -> [w270]
              stop <- w267 stop-if-true
              n277 = xnode "读取/写入控件"("FPGA VI引用输入"=w270) -> ("stop"=w269:bool)  [unwired: 1 in, 2 out]
              n278 = local read "stop"() -> (w268:bool)
              n279 = Wait (ms)(milliseconds to wait=u32 10 ("等待时间（毫秒）")) -> ()  [unwired: 1 out]
              n280 = Or(x=w269, y=w268) -> (x .or. y?=w267:bool)
            }
          }
          frame #1 {
            n281 = local write "TM state"("Idle" ("TM state")) -> ()
            n282 = local write "running"(FALSE ("running")) -> ()
            n283 = local write "stop"(TRUE ("stop")) -> ()
          }
        }
        n284 = while {
          shift-right: [w242] -> _
          shift-left: _ -> [w244]
          stop <- w246 stop-if-true
          n285 = local read "TM state"() -> (w242:string)
          n286 = Not Equal?(x=w244, y=w242) -> (x != y?=w243:bool)
          n287 = case shown="真" w243 {
            tunnel: w242 -> [_ w247]
            frame False {
            }
            frame True {
              n288 = case shown="\"running\"" w247 {
                frame "Idle", Default {
                  n289 = shared-variable "我的电脑\\NTM Epics server.lvlib\\ST:TM4:STATE"(0 ("ST:TM4:STATE")) -> ()  [unwired: 1 in, 1 out]
                }
                frame "Ready" {
                  n290 = shared-variable "我的电脑\\NTM Epics server.lvlib\\ST:TM4:STATE"(2 ("ST:TM4:STATE")) -> ()  [unwired: 1 in, 1 out]
                }
                frame "running" {
                  n291 = shared-variable "我的电脑\\NTM Epics server.lvlib\\ST:TM4:STATE"(15 ("ST:TM4:STATE")) -> ()  [unwired: 1 in, 1 out]
                }
              }
            }
          }
          n292 = Wait (ms)(milliseconds to wait=u32 100 ("等待时间（毫秒）")) -> ()  [unwired: 1 out]
          n293 = local read "stop"() -> (w246:bool)
        }
      }
    }
    n294 = local read "lvht 1"() -> ()  [unwired: 1 out]
    n295 = Current VI's Path() -> (path=w225:path)
    n296 = Strip Path(path=w225) -> (stripped path=w224:path)  [unwired: 1 out]
    n297 = constructor class="NewTmMdsSaveLoder"() -> (reference out=w209:refnum<k24>)  [unwired: 3 in, 2 out]
    n298 = Build Path(base path=w224, name or relative path="mdsplus" ("名称或相对路径")) -> (appended path=w222:path)
    n299 = local read "hr 1"() -> ()  [unwired: 1 in]
    n300 = Open/Create/Replace File(file path (use dialog)=w222, operation (0:open)=T7."replace or create" ("操作(0:open)")) -> (refnum out=w220:refnum<file>)  [unwired: 4 in, 2 out]
    n301 = local read "title"() -> (w219:string[])
    n302 = Write to Binary File(file (use dialog)=w220, data=w219) -> (refnum out=w214:refnum<file>)  [unwired: 4 in, 2 out]
    n303 = local read "act"() -> (w218:bool[])
    n304 = Write to Binary File(file (use dialog)=w214, data=w218) -> (refnum out=w213:refnum<file>)  [unwired: 4 in, 2 out]
    n305 = local read "start"() -> (w217:dbl[])
    n306 = Write to Binary File(file (use dialog)=w213, data=w217) -> (refnum out=w212:refnum<file>)  [unwired: 4 in, 2 out]
    n307 = local read "lenght"() -> (w216:dbl[])
    n308 = Write to Binary File(file (use dialog)=w212, data=w216) -> (refnum out=w211:refnum<file>)  [unwired: 4 in, 2 out]
    n309 = local read "detail"() -> (w215:string[])
    n310 = Write to Binary File(file (use dialog)=w211, data=w215) -> (refnum out=w210:refnum<file>)  [unwired: 4 in, 2 out]
    n311 = Close File(refnum=w210) -> (path=w208:path)  [unwired: 1 in, 1 out]
    n312 = Path To String(path=w208) -> (string=w207:string)
    n313 = invoke on="调用节点" class="NewTmMdsSaveLoder" method="UploadToMds"(reference=w209, "filePath"=w207) -> ()  [unwired: 6 in, 8 out]
  }
